vi "Transform.vi"() -> ()   [LabVIEW 2024]
uses:
  <vilib>/Utility/file.llb/Write Delimited Spreadsheet (DBL).vi
panel:
  out "data":dbl[](array[numeric])
  in  "Path":path
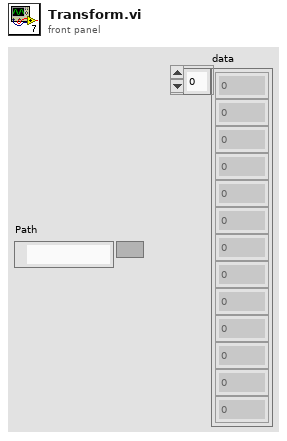
[diagram p1: front panel]
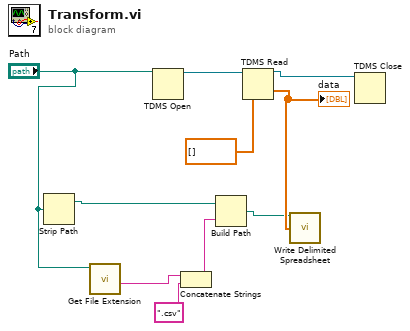
[diagram p0: block diagram]
diagram:
  n1 = Strip Path(path="Path") -> (stripped path=w6:path)  [unwired: 1 out]
  n2 = call <vilib>:"Get File Extension.vi"("file"="Path") -> ("filename without extension"=w3:string)  [unwired: 6 in, 4 out]
  n3 = TDMS Open(11:"Path") -> (3:w10:refnum<k34>)  [unwired: 6 in, 1 out]
  n4 = Concatenate Strings(w3, ".csv" ("string")) -> (w4:string)
  n5 = Build Path(base path=w6, name or relative path=w4) -> (appended path=w1:path)
  n6 = TDMS Read(0:w10, 12:dbl[] []) -> (4:w9:refnum<k34>, 10:w7:dbl[])  [unwired: 6 in, 4 out]
  "data" <- w7
  n7 = call-poly <vilib>:"Write Delimited Spreadsheet.vi"("file path (dialog if empty)"=w1, "1D data"=w7) -> ()  [unwired: 12 in, 2 out]
  n8 = TDMS Close(11:w9) -> ()  [unwired: 1 in, 2 out]
